vi "Set Mixer Printing Speed.vi"(8 "error in (no error)":errorcluster, 10 "Print Speed":dbl, 11 "Feeder Actor.lvlib:Mixer.lvclass":refnum<class "Mixer.lvclass">) -> (0 "error out":errorcluster, 3 "Feeder Actor.lvlib:Mixer.lvclass 2":refnum<class "Mixer.lvclass">)   [LabVIEW 2018, in "Feeder Actor.lvlib" / "Mixer.lvclass"]
uses:
  Mixer.lvclass
  Mixer.lvclass/Mixer.ctl
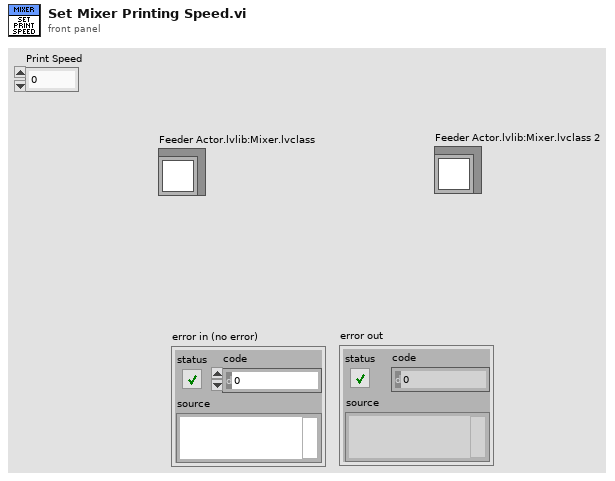
[diagram p1: front panel]
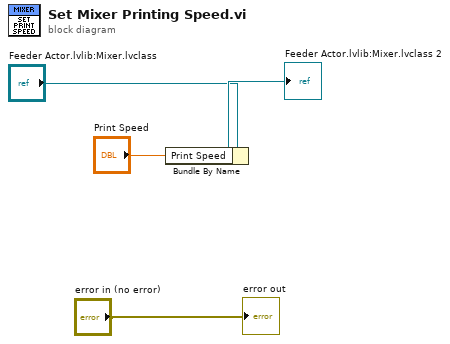
[diagram p0: block diagram]
diagram:
  n1 = Bundle By Name(cluster="Feeder Actor.lvlib:Mixer.lvclass", "Print Speed"="Print Speed") -> (→"Feeder Actor.lvlib:Mixer.lvclass 2":refnum<class "Mixer.lvclass">)
  "error out" <- "error in (no error)"
